vi "运维调试_总氮.vi"() -> ()   [LabVIEW 2016, in "斯坦道总氮.lvlib"]
uses:
  <vilib>/Utility/miscctls.llb/LVPointTypeDef.ctl
  <vilib>/Utility/config.llb/NI_LVConfig.lvlib
  <vilib>/ptbypt/NI_PtbyPt.lvlib
panel:
  out "一级权限":bool
  out "二级权限":bool
  out "输入密码":u32
  out "布尔":bool
  in  "流程固件":bool
  in  "仪器参数设置":bool
  in  "量程参数读取":T1
  in  "模块启用":bool
  in  "串口设置":bool
  in  "公式一键写入":bool
  in  "流程路径":path=path "C:/Users/STD/Documents/斯坦道流程文件/流程.xml"
  in  "曲线模型":cluster{"X^2":dbl, "X":dbl, "B":dbl}(xcontrol)
  out "字符串":string
  in  "质控参数设置":bool
  in  "自动测试量程配置":T2
  out "温度2":sgl
  out "温度1":sgl
  out "ADC":sgl
  out "固件版本号":string
  in  "数组":string[](array[string])
  in  "量程切换阈值写入":bool
  in  "量程切换阈值读取":bool
  in  "参数下拉列表":enum16{"总磷", "总氮"}(ring)=enum."总氮"
  in  "量程下拉列表":enum16{"低量程", "高量程"}(ring)
  in  "测量模式下拉列表":enum16{"水样测量", "零点核查", "跨度核查", "标样核查", "加标回收"}(ring)
  in  "公式":cluster{"X^2":dbl, "X":dbl, "b":dbl}
  in  "写公式":bool
  in  "读公式":bool
  in  "返回":bool
  in  "设置":bool
  out "序列号":string="序列号"
  out "测量数据":T3(xcontrol)
  out "集成报警信息":string
  out "定时启动":bool
  out "总磷总氮运行状态":T4(xcontrol)
  in  "停止":bool
  in  "手动启动":bool
  in  "单步测试":bool
  in  "总磷氨氮调试":u16[](xcontrol)
  out "F3":sgl format="%#.6f"
  out "F2":sgl format="%#.6f"
  out "F1":sgl format="%#.6f"
  out "F0":sgl format="%#.6f"
  out "多列列表框":i32(listbox)
  # "参数设置"
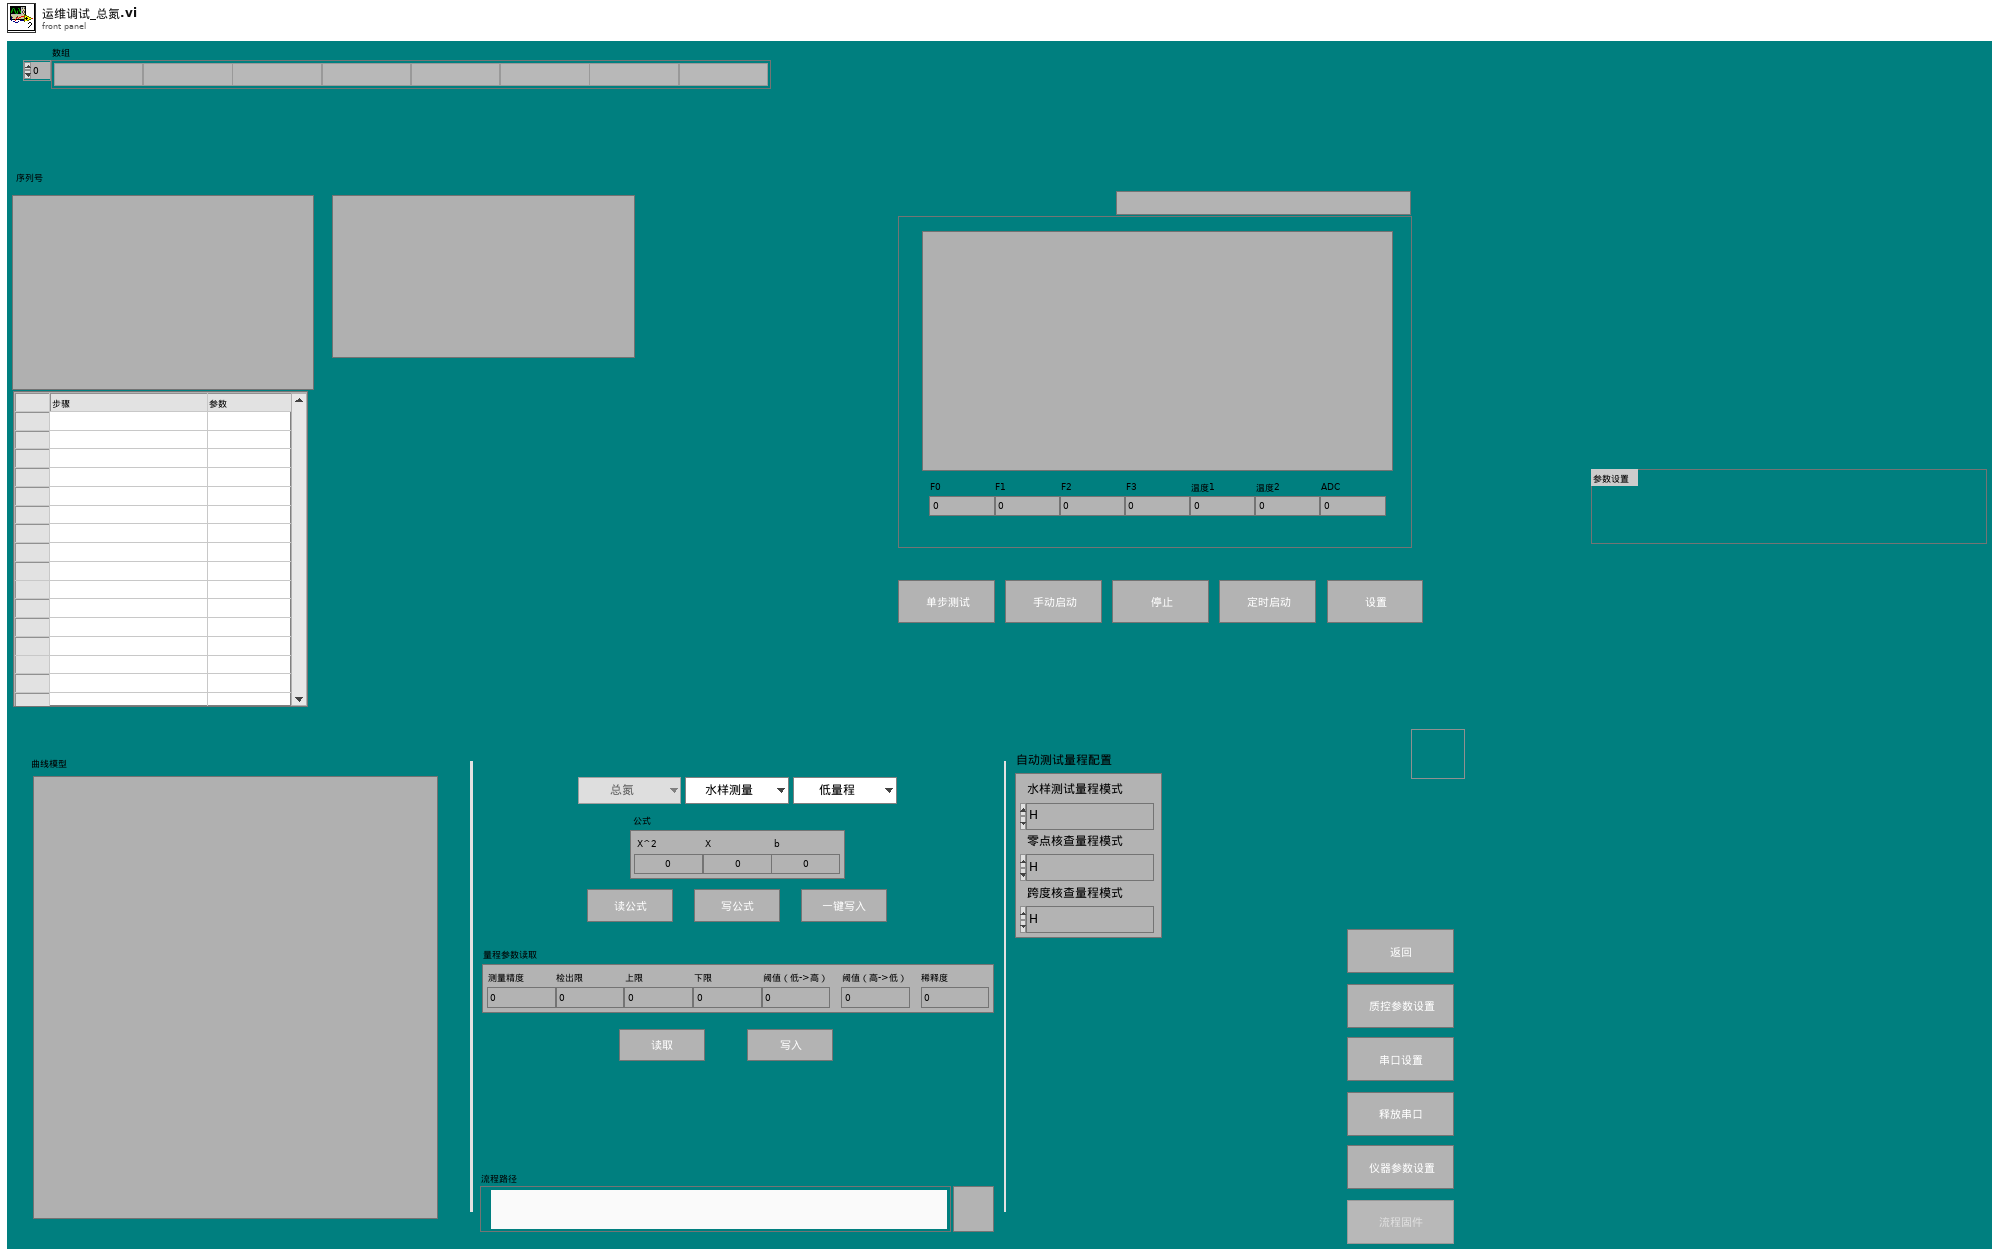
[diagram p1: front panel]
types:
  T1 = cluster{"测量精度":dbl, "检出限":dbl, "上限":dbl, "下限":dbl, "阈值（低->高）":dbl, "阈值（高->低）":dbl, "稀释度":dbl}
  T2 = cluster{"水样测试量程模式":enum16{"H", "L", "AUTO"}, "空白核查量程模式":enum16{"H", "L", "AUTO"}, "跨度核查量程模式":enum16{"H", "L", "AUTO"}}
  T3 = cluster{"flowid":u16, "测量精度":u16, "测量数据区":cluster{"因子编码":u32, "单位":u16, "标样参考值":sgl, "水样数据时间":timestamp, "水样实测值":sgl, "水样数据标识":string, "标样数据时间":timestamp, "标样实测值":sgl, "标样数据标识":string, "空白数据时间":timestamp, "空白实测值":sgl, "空白数据标识":string, "零点核查数据时间":timestamp, "零点核查实测值":sgl, "零点核查数据标识":string, "跨度核查数据时间":timestamp, "跨度核查实测值":sgl, "跨度核查数据标识":string, "加标回收数据时间":timestamp, "加标回收实测值":sgl, "加标回收数据标识":string, "平行样数据时间":timestamp, "平行样实测值":sgl, "平行样数据标识":string, "F0":sgl, "F1":sgl, "F2":sgl, "F3":sgl, "F4":sgl, "F5":sgl, "F6":sgl, "F7":sgl, "温度":sgl, "湿度":sgl, "X值":sgl, "fidrange":sgl}}
  T4 = cluster{"系统时间":timestamp, "工作状态":enum16{"空闲", "水样测试", "标样核查", "零点核查", "跨度核查", "空白测试", "平行样测试", "加标回收", "空白校准", "标样校准", "初始化（清洗）"}, "测量模式":enum16{"待机", "连续模式", "周期模式", "定点模式", "受控模式", "手动模式"}, "告警代码":u16, "故障代码":u16, "日志代码":u16, "软件版本":u16, "F0":sgl, "F1":sgl, "F2":sgl, "F3":sgl, "T":sgl, "H":sgl, "id":u16, "flowid":u16, "量程":u16, "总磷控温温度1":sgl, "营养盐控温温度2":sgl, "ADC":sgl}
  T5 = enum16{"启动测量", "标样核查", "零点核查", "跨度核查", "空白测试", "平行样测试", "加标回收", "空白校准", "标样校准", "初始化（清洗）", "停止测试", "仪器重启", "校时", "模式设置", "测量间隔设置"}
  T6 = cluster{"控制命令":enum16{"启动测量", "标样核查", "零点核查", "跨度核查", "空白测试", "平行样测试", "加标回收", "空白校准", "标样校准", "初始化（清洗）", "停止测试", "仪器重启", "校时", "模式设置", "测量间隔设置"}, "周期设置类型":enum16{"定点启动", "间隔启动"}, "定时功能启用":bool, "定时间隔":dbl, "24H周期设置":bool[], "零点核查时间":u16, "跨度核查时间":u16, "质控频次":enum16{"关闭", "每天", "星期一", "星期二", "星期三", "星期四", "星期五", "星期六", "星期日"}}
  T7 = enum16{"关闭", "每天", "星期一", "星期二", "星期三", "星期四", "星期五", "星期六", "星期日"}
  T8 = typedef "LVDateTimeRec.ctl" = cluster{"秒数的小数部分":dbl, "秒":i32, "分":i32, "时":i32, "日":i32, "月":i32, "年":i32, "天数（周）":i32, "天数（年）":i32, "DST":i32}
  T9 = enum16{"空闲", "水样测试", "标样核查", "零点核查", "跨度核查", "空白测试", "平行样测试", "加标回收", "空白校准", "标样校准", "初始化（清洗）"}
  T10 = enum32{"Bad", "Idle", "Run top level", "Running"}
  T11 = typedef "LVPointTypeDef.ctl" = cluster{"Horizontal":i16, "Vertical":i16}
  T12 = cluster{"因子编码":u32, "单位":u16, "标样参考值":sgl, "水样数据时间":timestamp, "水样实测值":sgl, "水样数据标识":string, "标样数据时间":timestamp, "标样实测值":sgl, "标样数据标识":string, "空白数据时间":timestamp, "空白实测值":sgl, "空白数据标识":string, "零点核查数据时间":timestamp, "零点核查实测值":sgl, "零点核查数据标识":string, "跨度核查数据时间":timestamp, "跨度核查实测值":sgl, "跨度核查数据标识":string, "加标回收数据时间":timestamp, "加标回收实测值":sgl, "加标回收数据标识":string, "平行样数据时间":timestamp, "平行样实测值":sgl, "平行样数据标识":string, "F0":sgl, "F1":sgl, "F2":sgl, "F3":sgl, "F4":sgl, "F5":sgl, "F6":sgl, "F7":sgl, "温度":sgl, "湿度":sgl, "X值":sgl, "fidrange":u16}
  T13 = typedef "NI_LVConfig.lvlib/Config Data RefNum.ctl" = refnum<k1>
  T14 = enum8{"Enabled", "Disabled", "Disabled and Grayed Out"}
  T15 = cluster{"启动模式":enum16{"跨度核查", "水样测量", "空白核查", "标样核查", "加标回收"}, "启动参数":u16, "量程":enum16{"低量程", "高量程"}}
  T16 = cluster{"时间标识":timestamp, "设备":string, "日志信息":string, "流程参数":string}
  T17 = cluster{"时间标识":timestamp, "设备":string, "日志信息":string}
  T18 = typedef "LVRowAndColumnUnsignedTypeDef.ctl" = cluster{"Row":u32, "Column":u32}
  T19 = cluster{"参数下拉列表":enum16{"总磷", "总氮"}, "测量模式下拉列表":enum16{"水样测量", "零点核查", "跨度核查", "标样核查", "加标回收"}, "量程下拉列表":enum16{"低量程", "高量程"}}
  T20 = cluster{"站号":u16, "量程切换":enum32{"H", "L", "AUTO"}, "控制命令":enum16{"启动测量", "标样核查", "零点核查", "跨度核查", "空白测试", "平行样测试", "加标回收", "空白校准", "标样校准", "初始化（清洗）", "停止测试", "仪器重启", "校时", "模式设置", "测量间隔设置"}, "模式设置":enum16{"待机", "连续模式", "周期模式", "定点模式", "受控模式", "手动模式"}, "测量间隔":u16}
  T21 = cluster{"跨度值":dbl, "零点标准液浓度":dbl, "跨度标准液浓度":dbl, "标准液标准浓度":dbl}
  T22 = cluster{"确定":bool, "跨度值":dbl, "零点标准液浓度":dbl, "跨度标准液浓度":dbl, "标准液标准浓度":dbl}
  T23 = cluster{"测量量程":dbl, "测量精度":dbl, "测量间隔":dbl, "消解温度":dbl, "消解时长":dbl, "空白校准时间":timestamp, "曲线截距":dbl, "曲线斜率":dbl, "测量检出限":dbl, "测量信号值":dbl, "线性相关系数":dbl, "二次多项式系数":dbl, "标样校准时间":timestamp, "单位":u16}
  T24 = cluster{"确定":bool, "测量量程":dbl, "测量精度":dbl, "测量间隔":dbl, "消解温度":dbl, "消解时长":dbl, "空白校准时间":timestamp, "曲线截距":dbl, "曲线斜率":dbl, "测量检出限":dbl, "测量信号值":dbl, "线性相关系数":dbl, "二次多项式系数":dbl, "标样校准时间":timestamp, "单位":u16}
  T25 = cluster{"控制命令":enum16{"启动测量", "标样核查", "零点核查", "跨度核查", "空白测试", "平行样测试", "加标回收", "空白校准", "标样校准", "初始化（清洗）", "停止测试", "仪器重启", "校时", "模式设置", "测量间隔设置"}, "周期设置类型":enum16{"定点启动", "间隔启动"}, "定时功能启用":bool, "定时间隔":dbl, "24H周期设置":bool[], "空白核查时间":u16, "跨度核查时间":u16, "质控频次":enum16{"关闭", "每天", "星期一", "星期二", "星期三", "星期四", "星期五", "星期六", "星期日"}}
  T26 = cluster{"测量精度":u16, "检出限":dbl, "上限":dbl, "下限":dbl, "阈值（低->高）":dbl, "阈值（高->低）":dbl, "稀释度":dbl}
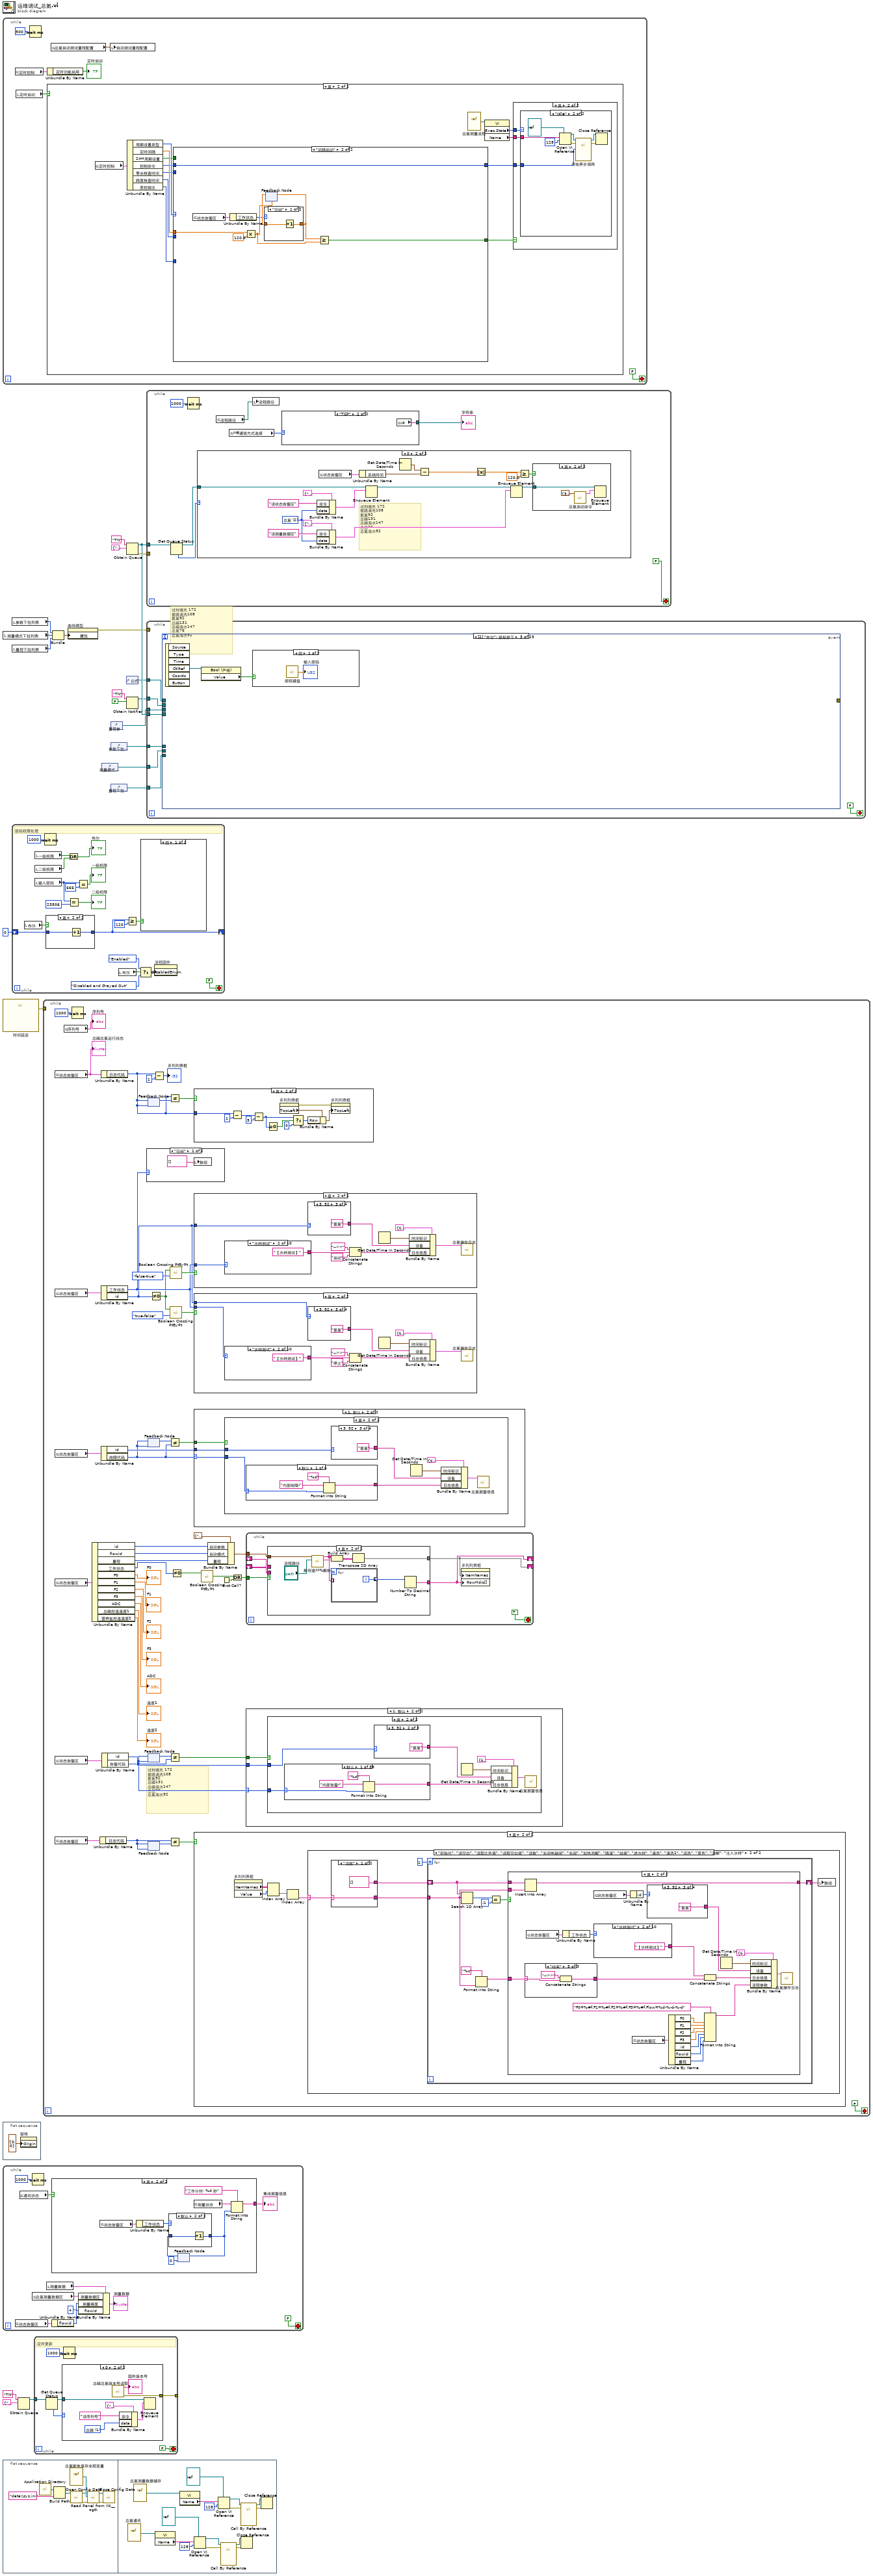
[diagram p0: block diagram]
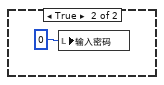
[diagram p2: hidden frame]
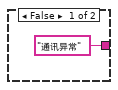
[diagram p5: hidden frame]
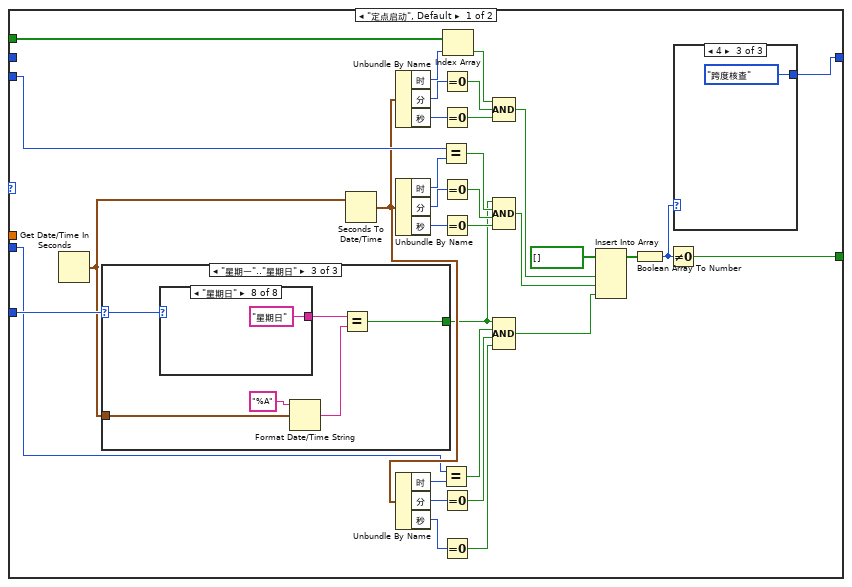
[diagram p8: hidden frame]
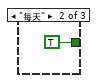
[diagram p10: hidden frame]
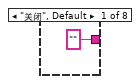
[diagram p11: hidden frame]
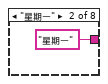
[diagram p12: hidden frame]
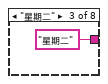
[diagram p13: hidden frame]
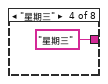
[diagram p14: hidden frame]
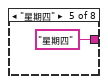
[diagram p15: hidden frame]
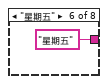
[diagram p16: hidden frame]
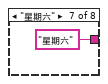
[diagram p17: hidden frame]
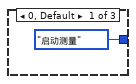
[diagram p18: hidden frame]
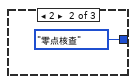
[diagram p19: hidden frame]
diagram:
  # "试剂填充 172 \n管路清洗108\n氨氮92\n总磷131\n总磷海水147\n总氮76\n总氮海水92"
  n1 = while {
    stop <- FALSE stop-if-true
    n2 = global read "总氮断电保存全局变量.vi" "定时控制"() -> (w24:T6)
    n3 = local read "定时启动"() -> (w26:bool)
    n4 = Wait (ms)(milliseconds to wait=u32 500 ("等待时间（毫秒）")) -> ()  [unwired: 1 out]
    n5 = Unbundle By Name(w24) -> ("定时功能启用"=→"定时启动":bool)
    n6 = case shown="真" w26 {
      frame False {
      }
      frame True {
        n7 = global read "总氮断电保存全局变量.vi" "定时控制"() -> (w41:T6)
        n8 = Unbundle By Name(w41) -> ("周期设置类型"=w37:enum16{"定点启动", "间隔启动"}, "定时间隔"=w36:dbl, "24H周期设置"=w35:bool[], "控制命令"=w34:T5, "零点核查时间"=w31:u16, "跨度核查时间"=w30:u16, "质控频次"=w29:T7)
        n9 = case shown="\"间隔启动\"" w37 {
          tunnel: w36 -> [_ w99]
          tunnel: w35 -> [w65 _]
          tunnel: [w43 w97] -> w32
          tunnel: w34 -> [_ w95]
          tunnel: [w69 w95] -> w33
          tunnel: w29 -> [w68 _]
          tunnel: w31 -> [w61 _]
          tunnel: w30 -> [w50 _]
          frame "定点启动", Default {
            n10 = Get Date/Time In Seconds() -> (seconds since 1Jan1904=w67:timestamp)
            n11 = case shown="\"星期一\"..\"星期日\"" w68 {
              selector: w68 -> [_ _ w79]
              tunnel: w67 -> [_ _ w80]
              tunnel: [_ TRUE w76] -> w49
              frame "关闭", Default {
              }
              frame "每天" {
              }
              frame "星期一".."星期日" {
                n12 = case shown="\"星期日\"" w79 {
                  tunnel: ["" ("时间格式字符串(%c)") "星期一" ("时间格式字符串(%c)") "星期二" ("时间格式字符串(%c)") "星期三" ("时间格式字符串(%c)") "星期四" ("时间格式字符串(%c)") "星期五" ("时间格式字符串(%c)") "星期六" ("时间格式字符串(%c)") "星期日" ("时间格式字符串(%c)")] -> w78
                  frame "关闭", Default {
                  }
                  frame "星期一" {
                  }
                  frame "星期二" {
                  }
                  frame "星期三" {
                  }
                  frame "星期四" {
                  }
                  frame "星期五" {
                  }
                  frame "星期六" {
                  }
                  frame "星期日" {
                  }
                }
                n13 = Format Date/Time String(time format string (%c)="%A" ("时间格式字符串(%c)"), seconds (now)=w80) -> (date/time string=w77:string)  [unwired: 1 in]
                n14 = Equal?(x=w78, y=w77) -> (x = y?=w76:bool)
              }
            }
            n15 = Seconds To Date/Time(time stamp (now)=w67) -> (date time rec=w51:T8)  [unwired: 1 in]
            n16 = Unbundle By Name(w51) -> ("时"=w74:i32, "分"=w72:i32, "秒"=w73:i32)
            n17 = Unbundle By Name(w51) -> ("时"=w62:i32, "分"=w64:i32, "秒"=w63:i32)
            n18 = Unbundle By Name(w51) -> ("时"=w54:i32, "分"=w52:i32, "秒"=w53:i32)
            n19 = Equal?(x=w61, y=w62) -> (x = y?=w60:bool)
            n20 = Equal?(x=w50, y=w54) -> (x = y?=w55:bool)
            n21 = Equal To 0?(x=w72) -> (x = 0?=w71:bool)
            n22 = Equal To 0?(x=w73) -> (x = 0?=w70:bool)
            n23 = Equal To 0?(x=w64) -> (x = 0?=w59:bool)
            n24 = Equal To 0?(x=w63) -> (x = 0?=w58:bool)
            n25 = Equal To 0?(x=w52) -> (x = 0?=w56:bool)
            n26 = Equal To 0?(x=w53) -> (x = 0?=w57:bool)
            n27 = Index Array(array=w65, index=w74) -> (element=w66:bool)
            n28 = Compound Arithmetic op=AND ("复合运算")(w66, w71, w70) -> (w47:bool)
            n29 = Compound Arithmetic op=AND ("复合运算")(w49, w60, w59, w58) -> (w46:bool)
            n30 = Compound Arithmetic op=AND ("复合运算")(w49, w55, w56, w57) -> (w45:bool)
            n31 = Insert Into Array(array=bool[] [], new element #1=w47, new element #2=w46, new element #3=w45) -> (w44:bool[])  [unwired: 1 in]
            n32 = Boolean Array To Number(Boolean array=w44) -> (number=w42:u32)
            n33 = Not Equal To 0?(x=w42) -> (x != 0?=w43:bool)
            n34 = case shown="4" w42 {
              tunnel: [T5."启动测量" ("控制命令") T5."零点核查" ("控制命令") T5."跨度核查" ("控制命令")] -> w69
              frame 0, Default {
              }
              frame 2 {
              }
              frame 4 {
              }
            }
          }
          frame "间隔启动" {
            n35 = global read "VAR总氮全局变量.vi" "状态告警区"() -> (w94:T4)
            n36 = Unbundle By Name(w94) -> ("工作状态"=w93:T9)
            n37 = Multiply(x=w99, y=120.0) -> (x*y=w96:dbl)
            n38 = feedback #1(w96) -> (w101:dbl)
            n39 = case shown="\"空闲\"" w93 {
              tunnel: w101 -> [w103 _]
              tunnel: [w102 _] -> w100
              frame "空闲" {
                n40 = Increment(x=w103) -> (x+1=w102:dbl)
              }
              frame "水样测试", Default {
              }
            }
            n41 = feedback-in #1(w100) -> ()
            n42 = Greater Or Equal?(x=w100, y=w96) -> (x >= y?=w97:bool)
          }
        }
        n43 = vi-ref "总氮测量流程.vi"() -> (w40:refnum<vi>)
        n44 = property class="VI"(reference=w40) -> ("Exec.State"=w38:T10, "Name"=w39:string)  [unwired: 1 in, 2 out]
        n45 = case shown="真" w32 {
          tunnel: w39 -> [_ w106]
          tunnel: w33 -> [_ w105]
          tunnel: w38 -> [_ w104]
          frame False {
          }
          frame True {
            n46 = case shown="\"Idle\"" w104 {
              tunnel: w106 -> [_ w110]
              tunnel: w105 -> [_ w108]
              frame "Bad", Default {
              }
              frame "Idle" {
                n47 = Open VI Reference(type specifier VI Refnum (for type only)=refnum<vi> refnum, vi path=w110, options=128 ("选项")) -> (vi reference=w111:refnum<vi>, error out=w112:errorcluster)  [unwired: 3 in]
                n48 = call-by-ref "开始异步调用"(reference=w111, error in=w112, "控制命令"=w108) -> (reference out=w113:refnum<vi>, error out=w114:errorcluster)  [unwired: 11 in]
                n49 = Close Reference(reference=w113, error in (no error)=w114) -> ()  [unwired: 1 out]
              }
            }
          }
        }
      }
    }
    n50 = global read "总氮断电保存全局变量.vi" "总氮自动测试量程配置"() -> (w25:T2)
    n51 = local write "自动测试量程配置"(w25) -> ()
  }
  n52 = local read "测量模式下拉列表"() -> (w4:enum16{"水样测量", "零点核查", "跨度核查", "标样核查", "加标回收"})
  n53 = call "时间延迟"() -> ("error out"=w14:errorcluster)  [unwired: 11 in]
  n54 = flat-sequence {
    frame #0 {
      n55 = property on="窗格" class="Pane"("Origin"=T11 {"Horizontal"=0, "Vertical"=0} ("原点")) -> ()  [unwired: 2 in, 2 out]
    }
  }
  n56 = while {
    stop <- FALSE stop-if-true
    n57 = global read "VAR总氮全局变量.vi" "状态告警区"() -> (w121:T4)
    n58 = global read "VAR总氮全局变量.vi" "通讯状态"() -> (w123:bool)
    n59 = Wait (ms)(milliseconds to wait=u32 1000 ("等待时间（毫秒）")) -> ()  [unwired: 1 out]
    n60 = global read "VAR总氮全局变量.vi" "总氮测量数据区"() -> (w117:T12)
    n61 = local read "测量数据"() -> (w116:T3)
    n62 = case shown="真" w123 {
      tunnel: ["通讯异常" ("集成报警信息") w128] -> w122
      frame False {
      }
      frame True {
        n63 = global read "VAR总氮全局变量.vi" "状态告警区"() -> (w134:T4)
        n64 = Unbundle By Name(w134) -> ("工作状态"=w133:T9)
        n65 = feedback #2(0) -> (w131:i32)
        n66 = case shown="默认" w133 {
          tunnel: w131 -> [_ w136]
          tunnel: [_ w135] -> w129
          frame "空闲" {
          }
          frame Default {
            n67 = Increment(x=w136) -> (x+1=w135:i32)
          }
        }
        n68 = feedback-in #2(w129) -> ()
        n69 = global read "VAR总氮全局变量.vi" "测量状态"() -> (w127:string)
        n70 = Format Into String(format string="工作计时: %d 秒" ("格式字符串"), initial string=w127, w129) -> (resulting string=w128:string)  [unwired: 1 in, 1 out]
      }
    }
    "集成报警信息" <- w122
    n71 = Unbundle By Name(w121) -> ("flowid"=w120:u16)
    n72 = Bundle By Name(cluster=w116, "测量数据区"=w117, "测量精度"=u16 4, "flowid"=w120) -> (→"测量数据":T3)
  }
  n73 = flat-sequence {
    frame #0 {
      n74 = call <vilib>:"Application Directory.vi"() -> ("Application Directory"=w144:path)
      n75 = Build Path(base path=w144, name or relative path="data\\sys.ini" ("名称或相对路径")) -> (appended path=w142:path)
      n76 = vi-ref "总氮断电保存全局变量.vi"() -> (w140:refnum<vi>)
      n77 = call <vilib>:"Open Config Data.vi"("configuration file path"=w142) -> ("error out"=w138:errorcluster, "refnum"=w141:T13)  [unwired: 8 in, 1 out]
      n78 = call <userlib>:"Read Panel from INI__ogtk.vi"("error in (no error)"=w138, "VI ref"=w140, "refnum"=w141) -> ("error out"=w137:errorcluster, "refnum out"=w139:T13)  [unwired: 7 in]
      n79 = call <vilib>:"Close Config Data.vi"("error in (no error)"=w137, "refnum"=w139) -> ()  [unwired: 8 in, 2 out]
    }
    frame #1 {
      n80 = vi-ref "总氮通讯.vi"() -> (w160:refnum<vi>)
      n81 = vi-ref "总氮测量数据储存.vi"() -> (w152:refnum<vi>)
      n82 = property class="VI"(reference=w160) -> ("Name"=w159:string)  [unwired: 1 in, 2 out]
      n83 = property class="VI"(reference=w152) -> ("Name"=w145:string)  [unwired: 1 in, 2 out]
      n84 = Open VI Reference(type specifier VI Refnum (for type only)=refnum<vi> refnum, vi path=w159, options=128 ("选项")) -> (vi reference=w157:refnum<vi>, error out=w155:errorcluster)  [unwired: 3 in]
      n85 = Open VI Reference(type specifier VI Refnum (for type only)=refnum<vi> refnum, vi path=w145, options=128 ("选项")) -> (vi reference=w147:refnum<vi>, error out=w149:errorcluster)  [unwired: 3 in]
      n86 = call-by-ref "?"(reference=w157, error in=w155) -> (reference out=w153:refnum<vi>, error out=w154:errorcluster)  [unwired: 12 in]
      n87 = call-by-ref "?"(reference=w147, error in=w149) -> (reference out=w151:refnum<vi>, error out=w150:errorcluster)  [unwired: 12 in]
      n88 = Close Reference(reference=w153, error in (no error)=w154) -> ()  [unwired: 1 out]
      n89 = Close Reference(reference=w151, error in (no error)=w150) -> ()  [unwired: 1 out]
    }
  }
  n90 = local read "参数下拉列表"() -> (w5:enum16{"总磷", "总氮"})
  n91 = local read "量程下拉列表"() -> (w3:enum16{"低量程", "高量程"})
  n92 = while {
    shift-right: [w167] -> _
    shift-left: u32 0 ("等待时间（毫秒）") -> [w168]
    stop <- FALSE stop-if-true
    # "密码权限处理"
    n93 = local read "布尔"() -> (w169:bool)
    n94 = local read "一级权限"() -> (w171:bool)
    n95 = local read "二级权限"() -> (w172:bool)
    n96 = local read "输入密码"() -> (w175:u32)
    n97 = Wait (ms)(milliseconds to wait=u32 1000 ("等待时间（毫秒）")) -> ()  [unwired: 1 out]
    n98 = case shown="真" w169 {
      tunnel: w168 -> [_ w182]
      tunnel: [_ w181] -> w167
      frame False {
      }
      frame True {
        n99 = Increment(x=w182) -> (x+1=w181:u32)
      }
    }
    n100 = Or(x=w171, y=w172) -> (x .or. y?=→"布尔":bool)
    n101 = Equal?(x=w175, y=u32 23506) -> (x = y?=→"二级权限":bool)
    n102 = Equal?(x=w175, y=u32 666) -> (x = y?=→"一级权限":bool)
    n103 = local read "布尔"() -> (w164:bool)
    n104 = Greater Or Equal?(x=w167, y=u32 120) -> (x >= y?=w165:bool)
    n105 = Select(t=T14."Enabled" ("禁用"), s=w164, f=T14."Disabled and Grayed Out") -> (s? t:f=w162:T14)
    n106 = case shown="假" w165 {
      frame False {
      }
      frame True {
        n107 = local write "输入密码"(u32 0 ("输入密码")) -> ()
      }
    }
    n108 = property on="流程固件" class="Bool"("DisabledEnum"=w162) -> ()  [unwired: 2 in, 2 out]
  }
  n109 = Obtain Queue(name (unnamed)="TN" ("名称（未命名）"), element data type=cluster{"命令":string, "data":variant} {"命令"="", "data"=variant}) -> (queue out=w11:refnum<queue>)  [unwired: 3 in, 2 out]
  n110 = while {
    tunnel: w11 -> [w187]
    tunnel: [w185] -> _
    stop <- FALSE stop-if-true
    # "定时更新"
    n111 = Get Queue Status(queue=w187) -> (queue out=w184:refnum<queue>, # elements in queue=w183:i32)  [unwired: 2 in, 6 out]
    n112 = case shown="0" w183 {
      tunnel: [_ w190] -> w185
      tunnel: w184 -> [_ w189]
      frame Default {
      }
      frame 0 {
        w193 = u16 1 items=["总磷"=1, "氨氮"=3] ("站号")
        n113 = call "总磷总氮版本号读取.vi"() -> ("error out"=w190:errorcluster, "固件版本号"=→"固件版本号":string)  [unwired: 10 in]
        n114 = Bundle By Name(cluster=cluster{"命令":string, "data":variant} {"命令"="", "data"=variant} ("元素"), "命令"="读序列号", "data"=w193) -> (w192:cluster{"命令":string, "data":variant})
        n115 = Enqueue Element(queue=w189, element=w192) -> ()  [unwired: 2 in, 3 out]
      }
    }
    n116 = Wait (ms)(milliseconds to wait=u32 1000 ("等待时间（毫秒）")) -> ()  [unwired: 1 out]
  }
  n117 = while {
    tunnel: w14 -> [_]
    stop <- FALSE stop-if-true
    # "试剂填充 172 \n管路清洗108\n氨氮92\n总磷131\n总磷海水147\n总氮76\n总氮海水92"
    n118 = global read "VAR总氮全局变量.vi" "状态告警区"() -> (w229:T4)
    "总磷总氮运行状态" <- w229
    n119 = global read "VAR总氮全局变量.vi" "状态告警区"() -> (w216:T4)
    n120 = global read "VAR总氮全局变量.vi" "状态告警区"() -> (w221:T4)
    n121 = global read "VAR总氮全局变量.vi" "状态告警区"() -> (w237:T4)
    n122 = global read "VAR总氮全局变量.vi" "状态告警区"() -> (w226:T4)
    n123 = global read "VAR总氮全局变量.vi" "状态告警区"() -> (w214:T4)
    n124 = global read "VAR总氮全局变量.vi" "序列号"() -> (→"序列号":string)
    n125 = Wait (ms)(milliseconds to wait=u32 1000 ("等待时间（毫秒）")) -> ()  [unwired: 1 out]
    n126 = Unbundle By Name(w237) -> ("id"=w234:u16, "flowid"=w236:u16, "量程"=w235:u16, "工作状态"=w204:T9, "F0"=→"F0":sgl, "F1"=→"F1":sgl, "F2"=→"F2":sgl, "F3"=→"F3":sgl, "ADC"=→"ADC":sgl, "总磷控温温度1"=→"温度1":sgl, "营养盐控温温度2"=→"温度2":sgl)
    n127 = Unbundle By Name(w214) -> ("日志代码"=w213:u16)
    n128 = Unbundle By Name(w229) -> ("日志代码"=w210:u16)
    n129 = Unbundle By Name(w216) -> ("工作状态"=w200:T9, "id"=w199:u16)
    n130 = Unbundle By Name(w221) -> ("id"=w220:u16, "故障代码"=w217:u16)
    n131 = Unbundle By Name(w226) -> ("id"=w225:u16, "告警代码"=w222:u16)
    n132 = case shown="\"空闲\"" w200 {
      frame "空闲" {
        n133 = local write "数组"(string[] [] ("数组")) -> ()
      }
      frame "水样测试", Default {
      }
    }
    n134 = feedback-in #3(w210) -> ()
    n135 = feedback #3(w210) -> (w242:u16)
    n136 = feedback #4(w217) -> (w218:u16)
    n137 = feedback-in #4(w217) -> ()
    n138 = feedback #5(w222) -> (w223:u16)
    n139 = feedback-in #5(w222) -> ()
    n140 = feedback #6(w213) -> (w215:u16)
    n141 = feedback-in #6(w213) -> ()
    n142 = Not Equal To 0?(x=w199) -> (x != 0?=w197:bool)
    n143 = Subtract(x=w210, y=1) -> (x-y=→"多列列表框":i32)
    n144 = Not Equal?(x=w210, y=w242) -> (x != y?=w241:bool)
    n145 = Not Equal?(x=w218, y=w217) -> (x != y?=w219:bool)
    n146 = Not Equal?(x=w223, y=w222) -> (x != y?=w224:bool)
    n147 = Not Equal?(x=w213, y=w215) -> (x != y?=w212:bool)
    n148 = call <vilib>:"Boolean Crossing PtByPt.vi"("direction"=enum16{"either", "false-true", "true-false"}."false-true", "input"=w197) -> ("crossing"=w202:bool)  [unwired: 1 in]
    n149 = call <vilib>:"Boolean Crossing PtByPt.vi"("direction"=enum16{"either", "false-true", "true-false"}."true-false", "input"=w197) -> ("crossing"=w196:bool)  [unwired: 1 in]
    n150 = Not Equal To 0?(x=w204) -> (x != 0?=w239:bool)
    n151 = case shown="真" w241 {
      tunnel: w210 -> [_ w452]
      frame False {
      }
      frame True {
        n152 = Subtract(x=w452, y=1) -> (x-y=w450:i32)
        n153 = Subtract(x=w450, y=5) -> (x-y=w454:i32)
        n154 = Greater Or Equal To 0?(x=w454) -> (x >= 0?=w453:bool)
        n155 = property on="多列列表框" class="MCListbox (严格)"() -> (error out=w458:errorcluster, "TopLeft"=w459:T18)  [unwired: 2 in, 1 out]
        n156 = Select(t=w454, s=w453, f=0) -> (s? t:f=w455:i32)
        n157 = Bundle By Name(cluster=w459, "Row"=w455) -> (w460:T18)
        n158 = property on="多列列表框" class="MCListbox (严格)"(error in=w458, "TopLeft"=w460) -> ()  [unwired: 1 in, 2 out]
      }
    }
    n159 = case shown="真" w202 {
      tunnel: w199 -> [_ w270]
      tunnel: w200 -> [_ w269]
      frame False {
      }
      frame True {
        n160 = case shown="\"水样测试\"" w269 {
          tunnel: [_ "【水样测试】" ("字符串") "【标样核查】" ("字符串") "【零点核查】" ("字符串") "【跨度核查】" ("字符串") "【空白测试】" ("字符串") "【平行样测试】" ("字符串") "【加标回收】" ("字符串") "【空白校准】" ("字符串") "【标样校准】" ("字符串")] -> w275
          frame "空闲", Default {
          }
          frame "水样测试" {
          }
          frame "标样核查" {
          }
          frame "零点核查" {
          }
          frame "跨度核查" {
          }
          frame "空白测试" {
          }
          frame "平行样测试" {
          }
          frame "加标回收" {
          }
          frame "空白校准" {
          }
          frame "标样校准" {
          }
        }
        n161 = case shown="3, 92" w270 {
          tunnel: [_ "总磷" ("table输入") "氨氮" ("table输入") "总氮" ("table输入")] -> w272
          frame Default {
          }
          frame 1, 131 {
          }
          frame 3, 92 {
          }
          frame 2, 76 {
          }
        }
        n162 = Concatenate Strings("-->>" ("字符串"), w275, "启动" ("字符串")) -> (w276:string)
        n163 = Get Date/Time In Seconds() -> (seconds since 1Jan1904=w273:timestamp)
        n164 = Bundle By Name(cluster=T16 {"时间标识"=timestamp(0 s since 1904-01-01), "设备"="", "日志信息"="", "流程参数"=""} ("data in"), "时间标识"=w273, "设备"=w272, "日志信息"=w276) -> (w271:T16)
        n165 = call "总氮操作日志.vi"("data in"=w271) -> ()  [unwired: 11 in]
      }
    }
    n166 = case shown="真" w196 {
      tunnel: w199 -> [_ w248]
      tunnel: w200 -> [_ w247]
      frame False {
      }
      frame True {
        n167 = case shown="\"水样测试\"" w247 {
          tunnel: [_ "【水样测试】" ("字符串") "【标样核查】" ("字符串") "【零点核查】" ("字符串") "【跨度核查】" ("字符串") "【空白测试】" ("字符串") "【平行样测试】" ("字符串") "【加标回收】" ("字符串") "【空白校准】" ("字符串") "【标样校准】" ("字符串")] -> w253
          frame "空闲", Default {
          }
          frame "水样测试" {
          }
          frame "标样核查" {
          }
          frame "零点核查" {
          }
          frame "跨度核查" {
          }
          frame "空白测试" {
          }
          frame "平行样测试" {
          }
          frame "加标回收" {
          }
          frame "空白校准" {
          }
          frame "标样校准" {
          }
        }
        n168 = case shown="3, 92" w248 {
          tunnel: [_ "总磷" ("table输入") "氨氮" ("table输入") "总氮" ("table输入")] -> w250
          frame Default {
          }
          frame 1, 131 {
          }
          frame 3, 92 {
          }
          frame 2, 76 {
          }
        }
        n169 = Concatenate Strings("-->>" ("字符串"), w253, "停止" ("字符串")) -> (w254:string)
        n170 = Get Date/Time In Seconds() -> (seconds since 1Jan1904=w251:timestamp)
        n171 = Bundle By Name(cluster=T16 {"时间标识"=timestamp(0 s since 1904-01-01), "设备"="", "日志信息"="", "流程参数"=""} ("data in"), "时间标识"=w251, "设备"=w250, "日志信息"=w254) -> (w249:T16)
        n172 = call "总氮操作日志.vi"("data in"=w249) -> ()  [unwired: 11 in]
      }
    }
    n173 = case shown="1, 默认" w217 {
      selector: w217 -> [_ w357]
      tunnel: w220 -> [_ w358]
      tunnel: w219 -> [_ w356]
      frame 0 {
      }
      frame 1, Default {
        n174 = case shown="真" w356 {
          tunnel: w358 -> [_ w365]
          tunnel: w357 -> [_ w360]
          frame False {
          }
          frame True {
            n175 = case shown="默认" w360 {
              selector: w360 -> [w367 _ _ _ _ _]
              tunnel: [w366 "无故障" "电机故障" "温度故障" "通讯故障" "滴定故障"] -> w359
              frame Default {
                n176 = Format Into String(format string="%d" ("格式字符串"), initial string="内部故障-" ("工作状态"), w367) -> (resulting string=w366:string)  [unwired: 1 in, 1 out]
              }
              frame 0 {
              }
              frame 1 {
              }
              frame 2 {
              }
              frame 3 {
              }
              frame 4 {
              }
            }
            n177 = case shown="3, 92" w365 {
              tunnel: [_ "总磷" ("table输入") "氨氮" ("table输入") "总氮" ("table输入")] -> w361
              frame Default {
              }
              frame 1, 131 {
              }
              frame 3, 92 {
              }
              frame 2, 76 {
              }
            }
            n178 = Get Date/Time In Seconds() -> (seconds since 1Jan1904=w362:timestamp)
            n179 = Bundle By Name(cluster=T17 {"时间标识"=timestamp(0 s since 1904-01-01), "设备"="", "日志信息"=""} ("data in"), "时间标识"=w362, "设备"=w361, "日志信息"=w359) -> (w363:T17)
            n180 = call "总氮报警信息.vi"("data in"=w363) -> ()  [unwired: 10 in, 1 out]
          }
        }
      }
    }
    n181 = case shown="真" w212 {
      frame False {
      }
      frame True {
        n182 = property on="多列列表框" class="MCListbox (严格)"() -> ("ItemNames"=w292:string[][], "Value"=w293:i32)  [unwired: 2 in, 2 out]
        n183 = Index Array(array=w292, index (row)=w293) -> (element=w291:string[])  [unwired: 1 in]
        n184 = Index Array(array=w291) -> (element=w290:string)  [unwired: 1 in]
        n185 = case shown="\"初始化\", \"读空白\", \"读取比色值\", \"读取空白值\", \"读数\", \"关闭电磁阀\", \"关阀\", \"加热消解\", \"降温\", \"结束\", \"进水样\", \"清洗\", \"清洗1\", \"润洗\", \"显色\", \"消解\", \"注入水样\"" w290 {
          selector: w290 -> [_ w296]
          frame Default {
          }
          frame "初始化", "读空白", "读取比色值", "读取空白值", "读数", "关闭电磁阀", "关阀", "加热消解", "降温", "结束", "进水样", "清洗", "清洗1", "润洗", "显色", "消解", "注入水样" {
            n186 = case shown="\"读数\"" w296 {
              selector: w296 -> [w300 w302]
              tunnel: [w300 w302] -> w295
              tunnel: [string[] [] ("数组") "数组"] -> w294
              frame "读数" {
              }
              frame Default {
              }
            }
            n187 = for {
              N: 1 -> [_]
              tunnel: w295 -> [w304]
              shift-right: [w303] -> w297
              shift-left: w294 -> [w305]
              n188 = Search 1D Array(1D array=w305, element=w304) -> (index of element=w308:i32)  [unwired: 1 in]
              n189 = Format Into String(format string="%s" ("格式字符串"), w304) -> (resulting string=w309:string)  [unwired: 2 in, 1 out]
              n190 = Equal?(x=w308, y=-1) -> (x = y?=w306:bool)
              n191 = case shown="真" w306 {
                tunnel: w309 -> [_ w317]
                tunnel: w305 -> [w311 w321]
                tunnel: w304 -> [_ w320]
                tunnel: [w311 w319] -> w303
                frame False {
                }
                frame True {
                  n192 = Insert Into Array(array=w321, new element=w320) -> (w319:string[])  [unwired: 1 in]
                  n193 = case shown="\"结束\"" w317 {
                    selector: w317 -> [w346 w349 w352]
                    tunnel: [w346 w348 w351] -> w313
                    frame Default {
                    }
                    frame "初始化" {
                      n194 = Concatenate Strings("-->>" ("字符串"), w349) -> (w348:string)
                    }
                    frame "结束" {
                      n195 = Concatenate Strings("-->>" ("字符串"), w352) -> (w351:string)
                    }
                  }
                  n196 = global read "VAR总氮全局变量.vi" "状态告警区"() -> (w316:T4)
                  n197 = Unbundle By Name(w316) -> ("工作状态"=w315:T9)
                  n198 = global read "VAR总氮全局变量.vi" "状态告警区"() -> (w336:T4)
                  n199 = case shown="\"水样测试\"" w315 {
                    tunnel: [_ "【水样测试】" ("字符串") "【标样核查】" ("字符串") "【零点核查】" ("字符串") "【跨度核查】" ("字符串") "【空白测试】" ("字符串") "【平行样测试】" ("字符串") "【加标回收】" ("字符串") "【空白校准】" ("字符串") "【标样校准】" ("字符串")] -> w314
                    frame "空闲", Default {
                    }
                    frame "水样测试" {
                    }
                    frame "标样核查" {
                    }
                    frame "零点核查" {
                    }
                    frame "跨度核查" {
                    }
                    frame "空白测试" {
                    }
                    frame "平行样测试" {
                    }
                    frame "加标回收" {
                    }
                    frame "空白校准" {
                    }
                    frame "标样校准" {
                    }
                  }
                  n200 = Unbundle By Name(w336) -> ("id"=w335:u16)
                  n201 = global read "VAR总氮全局变量.vi" "状态告警区"() -> (w331:T4)
                  n202 = case shown="3, 92" w335 {
                    tunnel: [_ "总磷" ("table输入") "氨氮" ("table输入") "总氮" ("table输入")] -> w333
                    frame Default {
                    }
                    frame 1, 131 {
                    }
                    frame 3, 92 {
                    }
                    frame 2, 76 {
                    }
                  }
                  n203 = Unbundle By Name(w331) -> ("F0"=w328:sgl, "F1"=w327:sgl, "F2"=w326:sgl, "F3"=w325:sgl, "id"=w324:u16, "flowid"=w323:u16, "量程"=w322:u16)
                  n204 = Concatenate Strings(w314, w313) -> (w312:string)
                  n205 = Format Into String(format string="F0=%#f,F1=%#f,F2=%#f,F3=%#f,Flow=%d-%-d-%-d" ("格式字符串"), w328, w327, w326, w325, w324, w323, w322) -> (resulting string=w329:string)  [unwired: 2 in, 1 out]
                  n206 = Get Date/Time In Seconds() -> (seconds since 1Jan1904=w332:timestamp)
                  n207 = Bundle By Name(cluster=T16 {"时间标识"=timestamp(0 s since 1904-01-01), "设备"="", "日志信息"="", "流程参数"=""} ("data in"), "时间标识"=w332, "设备"=w333, "日志信息"=w312, "流程参数"=w329) -> (w334:T16)
                  n208 = call "总氮操作日志.vi"("data in"=w334) -> ()  [unwired: 11 in]
                }
              }
            }
            n209 = local write "数组"(w297) -> ()
          }
        }
      }
    }
    n210 = call <vilib>:"Boolean Crossing PtByPt.vi"("input"=w239) -> ("crossing"=w203:bool)  [unwired: 2 in]
    n211 = Bundle By Name(cluster=T15 {"启动模式"=enum."跨度核查", "启动参数"=1, "量程"=enum."低量程"} ("参数簇"), "启动参数"=w234, "启动模式"=w236, "量程"=w235) -> (w228:T15)
    n212 = First Call?() -> (First Call?: T/F=w240:bool)
    n213 = Or(x=w203, y=w240) -> (x .or. y?=w238:bool)
    n214 = while {
      tunnel: w238 -> [w438]
      tunnel: w228 -> [w437]
      shift-right: [w432] -> _
      shift-left: _ -> [w434]
      shift-right: [w433] -> _
      shift-left: _ -> [w435]
      stop <- TRUE stop-if-true
      n215 = case shown="真" w438 {
        tunnel: [w440 w448] -> w433
        tunnel: [w439 w447] -> w432
        tunnel: w437 -> [_ w442]
        tunnel: w435 -> [w440 _]
        tunnel: w434 -> [w439 _]
        frame False {
        }
        frame True {
          n216 = call "斯坦道XML解析.vi"("添加的路径"="流程路径", "参数簇"=w442) -> ("步骤时间"=w443:string[], "步骤名"=w445:string[])  [unwired: 8 in]
          n217 = Build Array(w445, w443) -> (w444:string[][])
          n218 = for {
            tunnel: w445 -> [_] mode=indexing
            tunnel: [w449] -> w446 mode=indexing
            i -> [w449]
          }
          n219 = Transpose 2D Array(2D array=w444) -> (transposed array=w447:string[][])
          n220 = Number To Decimal String(number=w446) -> (decimal integer string=w448:string[])  [unwired: 1 in]
        }
      }
      n221 = property on="多列列表框" class="MCListbox (严格)"("ItemNames"=w432, "RowHdrs[]"=w433) -> ()  [unwired: 2 in, 2 out]
    }
    n222 = case shown="1, 默认" w222 {
      selector: w222 -> [_ w379]
      tunnel: w225 -> [_ w380]
      tunnel: w224 -> [_ w378]
      frame 0 {
      }
      frame 1, Default {
        n223 = case shown="真" w378 {
          tunnel: w380 -> [_ w387]
          tunnel: w379 -> [_ w381]
          frame False {
          }
          frame True {
            n224 = case shown="默认" w381 {
              selector: w381 -> [w389 _ _ _ _ _ _ _ _ _ _ _ _ _ _ _ _ _ _ _ _ _ _ _ _ _ _ _ _ _ _ _ _ _ _ _ _ _]
              tunnel: [w388 "无告警" "缺试剂告警" "缺水样告警" "缺蒸馏水告警" "缺标液告警" "仪表漏液告警" "标定异常告警" "超量程告警" "加热异常" "低试剂预警" "超上限告警" "超下限告警" "仪表内部其他异常" "滴定异常告警" "电极异常告警" "量程切换告警" "参数设置告警" "PH电极电位异常" "电导率电极异常" "浊度光度异常" "溶解氧电极异常" "溶解氧光强异常" "温度异常告警" "PH异常告警" "溶解氧异常告警" "电导率异常告警" "浊度异常告警" "叶绿素异常告警" "藻密度异常告警" "蓝绿藻异常告警" "ORP异常告警" "氨氮异常告警" "清洁刷异常告警" "SD卡异常告警" "蓝牙异常告警" "WiFi异常告警" "流程异常告警"] -> w382
              frame Default {
                n225 = Format Into String(format string="%d" ("格式字符串"), initial string="内部告警-" ("工作状态"), w389) -> (resulting string=w388:string)  [unwired: 1 in, 1 out]
              }
              frame 0 {
              }
              frame 1 {
              }
              frame 2 {
              }
              frame 3 {
              }
              frame 4 {
              }
              frame 5 {
              }
              frame 6 {
              }
              frame 7 {
              }
              frame 8 {
              }
              frame 9 {
              }
              frame 10 {
              }
              frame 11 {
              }
              frame 12 {
              }
              frame 13 {
              }
              frame 14 {
              }
              frame 15 {
              }
              frame 16 {
              }
              frame 17 {
              }
              frame 18 {
              }
              frame 19 {
              }
              frame 20 {
              }
              frame 21 {
              }
              frame 22 {
              }
              frame 23 {
              }
              frame 24 {
              }
              frame 25 {
              }
              frame 26 {
              }
              frame 27 {
              }
              frame 28 {
              }
              frame 29 {
              }
              frame 30 {
              }
              frame 31 {
              }
              frame 32 {
              }
              frame 33 {
              }
              frame 34 {
              }
              frame 35 {
              }
              frame 36 {
              }
            }
            n226 = case shown="3, 92" w387 {
              tunnel: ["总磷" ("table输入") "氨氮" ("table输入") "总氮" ("table输入")] -> w383
              frame 1, 131 {
              }
              frame 3, 92 {
              }
              frame 2, 76, Default {
              }
            }
            n227 = Get Date/Time In Seconds() -> (seconds since 1Jan1904=w384:timestamp)
            n228 = Bundle By Name(cluster=T17 {"时间标识"=timestamp(0 s since 1904-01-01), "设备"="", "日志信息"=""} ("data in"), "时间标识"=w384, "设备"=w383, "日志信息"=w382) -> (w385:T17)
            n229 = call "总氮报警信息.vi"("data in"=w385) -> ()  [unwired: 10 in, 1 out]
          }
        }
      }
    }
  }
  n230 = Bundle("参数下拉列表"=w5, "测量模式下拉列表"=w4, "量程下拉列表"=w3) -> (w2:T19)  [unwired: 1 in]
  n231 = property on="曲线模型" class="曲线模型 (严格)"("属性"=w2) -> (error out=w10:errorcluster)  [unwired: 2 in, 1 out]
  n232 = control-ref of="测量模式下拉列表"() -> (w16:refnum<vi>)
  n233 = control-ref of="量程参数读取"() -> (w6:refnum<vi>)
  n234 = control-ref of="参数下拉列表"() -> (w17:refnum<vi>)
  n235 = control-ref of="量程下拉列表"() -> (w18:refnum<vi>)
  n236 = Obtain Queue(name (unnamed)="TN" ("名称（未命名）"), element data type=cluster{"命令":string, "data":variant} {"命令"="", "data"=variant}) -> (queue out=w19:refnum<queue>, error out=w20:errorcluster)  [unwired: 3 in, 1 out]
  n237 = control-ref of="公式"() -> (w15:refnum<vi>)
  n238 = Obtain Notifier(name (unnamed)="TN" ("名称（未命名）"), notification data type=FALSE) -> (notifier out=w7:refnum<notifier>)  [unwired: 2 in, 2 out]
  n239 = while {
    tunnel: w19 -> [w466]
    tunnel: w20 -> [_]
    stop <- FALSE stop-if-true
    n240 = Get Queue Status(queue=w466) -> (queue out=w462:refnum<queue>, # elements in queue=w461:i32)  [unwired: 2 in, 6 out]
    n241 = Wait (ms)(milliseconds to wait=u32 1000 ("等待时间（毫秒）")) -> ()  [unwired: 1 out]
    n242 = case shown="0" w461 {
      tunnel: w462 -> [_ w469]
      frame Default {
      }
      frame 0 {
        w478 = u16 2 items=["总磷"=1, "总氮"=2, "氨氮"=3] ("站号")
        # "试剂填充 172 \n管路清洗108\n氨氮92\n总磷131\n总磷海水147\n总氮76\n总氮海水92"
        n243 = Bundle By Name(cluster=cluster{"命令":string, "data":variant} {"命令"="", "data"=variant} ("元素"), "命令"="读状态告警区", "data"=w478) -> (w484:cluster{"命令":string, "data":variant})
        n244 = Bundle By Name(cluster=cluster{"命令":string, "data":variant} {"命令"="", "data"=variant} ("元素"), "命令"="读测量数据区", "data"=w478) -> (w481:cluster{"命令":string, "data":variant})
        n245 = global read "VAR总氮全局变量.vi" "状态告警区"() -> (w470:T4)
        n246 = Unbundle By Name(w470) -> ("系统时间"=w477:timestamp)
        n247 = Enqueue Element(queue=w469, element=w484) -> (queue out=w479:refnum<queue>)  [unwired: 2 in, 2 out]
        n248 = Get Date/Time In Seconds() -> (seconds since 1Jan1904=w476:timestamp)
        n249 = Subtract(x=w476, y=w477) -> (x-y=w475:dbl)
        n250 = Absolute Value(x=w475) -> (abs(x)=w474:dbl)
        n251 = Enqueue Element(queue=w479, element=w481) -> (queue out=w471:refnum<queue>)  [unwired: 2 in, 2 out]
        n252 = Greater Or Equal?(x=w474, y=120.0) -> (x >= y?=w472:bool)
        n253 = case shown="真" w472 {
          tunnel: w471 -> [_ w487]
          frame False {
          }
          frame True {
            n254 = call "总氮启动命令.vi"("参数"=T20 {"站号"=3, "量程切换"=enum."AUTO", "控制命令"=enum."校时", "模式设置"=enum."待机", "测量间隔"=0}) -> ("启动命令"=w486:cluster{"命令":string, "data":variant})  [unwired: 10 in]
            n255 = Enqueue Element(queue=w487, element=w486) -> ()  [unwired: 2 in, 3 out]
          }
        }
      }
    }
    n256 = global read "总氮断电保存全局变量.vi" "流程路径"() -> (w465:path)
    n257 = global read "总氮断电保存全局变量.vi" "MB通信方式选择"() -> (w463:enum16{"串口", "TCP"})
    n258 = local write "流程路径"(w465) -> ()
    n259 = case shown="\"TCP\"" w463 {
      tunnel: [w489 w490] -> w464
      frame "串口", Default {
        n260 = global read "总氮断电保存全局变量.vi" "VISA Resource"() -> (w489:refnum<visa-resource-name>)
      }
      frame "TCP" {
        n261 = global read "总氮断电保存全局变量.vi" "IP"() -> (w490:string)
      }
    }
    "字符串" <- w464
  }
  n262 = while {
    tunnel: w19 -> [w497]
    tunnel: w18 -> [w496]
    tunnel: w17 -> [w495]
    tunnel: w16 -> [w494]
    tunnel: w15 -> [w493]
    tunnel: w6 -> [w492]
    tunnel: w10 -> [_]
    tunnel: w7 -> [w491]
    stop <- FALSE stop-if-true
    n263 = event shown="[2] \"布尔\": 鼠标按下" {
      selector: _ -> [_ _ _ _ _ _ _ _ _ _ _ _ _ _ _ _ _ _ _ _ _ _ _]
      dyn-events: _ -> [_ _ _ _ _ _ _ _ _ _ _ _ _ _ _ _ _ _ _ _ _ _ _]
      timeout: _ -> [_ _ _ _ _ _ _ _ _ _ _ _ _ _ _ _ _ _ _ _ _ _ _]
      tunnel: w497 -> [_ _ _ _ w517 w545 _ _ _ _ _ _ w647 _ w672 w679 _ _ _ _ _ _ _]
      tunnel: w496 -> [_ _ _ _ _ _ _ _ _ _ _ _ _ _ _ _ _ _ _ w695 _ _ _]
      tunnel: w495 -> [_ _ _ _ _ _ _ _ _ _ _ _ _ _ _ _ _ _ _ w693 _ w711 w718]
      tunnel: w494 -> [_ _ _ _ _ _ _ _ _ _ _ _ _ _ _ _ _ _ _ w694 _ _ _]
      tunnel: w493 -> [_ _ _ _ _ _ _ _ _ _ _ _ _ _ _ _ _ _ _ w689 _ _ _]
      tunnel: w492 -> [_ _ _ _ _ _ _ _ _ _ _ _ _ _ _ _ _ _ _ _ _ w709 _]
      tunnel: w491 -> [_ _ _ _ _ _ _ _ _ _ _ _ _ _ _ w675 _ _ _ _ _ _ _]
      tunnel: [_ _ _ w503 _ _ _ _ _ _ _ _ _ _ _ _ _ _ _ _ _ _ _] -> _
      event Timeout {
        n264 = event-data() -> ()  [unwired: 1 in, 3 out]
      }
      event "流程固件": Value Change {
        n265 = event-data() -> ()  [unwired: 1 in, 6 out]
        n266 = call "流程固件设置对话框.vi"() -> ()  [unwired: 12 in]
      }
      event "布尔": Mouse Down {
        n267 = event-data() -> ("CtlRef"=w500:refnum<vi>)  [unwired: 1 in, 5 out]
        n268 = property class="Bool (严格)"(reference=w500) -> ("Value"=w499:bool)  [unwired: 1 in, 2 out]
        n269 = case shown="假" w499 {
          frame False {
            n270 = call "密码键盘.vi"() -> ("NewNumber"=→"输入密码":dbl)  [unwired: 1 in]
          }
          frame True {
            n271 = local write "输入密码"(u32 0 ("输入密码")) -> ()
          }
        }
      }
      event "测量模式下拉列表", "量程下拉列表", "参数下拉列表": Value Change {
        n272 = event-data() -> ()  [unwired: 1 in, 6 out]
        n273 = local read "测量模式下拉列表"() -> (w505:enum16{"水样测量", "零点核查", "跨度核查", "标样核查", "加标回收"})
        n274 = local read "参数下拉列表"() -> (w504:enum16{"总磷", "总氮"})
        n275 = local read "量程下拉列表"() -> (w506:enum16{"低量程", "高量程"})
        n276 = Bundle("参数下拉列表"=w504, "测量模式下拉列表"=w505, "量程下拉列表"=w506) -> (w507:T19)  [unwired: 1 in]
        n277 = property on="曲线模型" class="曲线模型 (严格)"("属性"=w507) -> (error out=w503:errorcluster)  [unwired: 2 in, 1 out]
      }
      event "串口设置": Value Change {
        n278 = event-data() -> ()  [unwired: 1 in, 6 out]
        n279 = global read "总氮断电保存全局变量.vi" "MB通信方式选择"() -> (w508:enum16{"串口", "TCP"})
        n280 = global read "总氮断电保存全局变量.vi" "VISA Resource"() -> (w514:refnum<visa-resource-name>)
        n281 = global read "总氮断电保存全局变量.vi" "PORT"() -> (w513:string)
        n282 = global read "总氮断电保存全局变量.vi" "IP"() -> (w509:string)
        n283 = call "串口配置.vi"("PORT"=w513, "IP"=w509, "MB通信方式选择"=w508, "请选择串口:"=w514) -> ("PORT 2"=w511:string, "IP 2"=w512:string, "确认 2"=w515:bool, "VISA资源名称 2"=w516:refnum<visa-resource-name>, "MB通信方式选择 2"=w510:enum16{"串口", "TCP"})  [unwired: 3 in]
        n284 = case shown="真" w515 {
          tunnel: w516 -> [_ w522]
          tunnel: w517 -> [_ w521]
          tunnel: w512 -> [_ w520]
          tunnel: w511 -> [_ w519]
          tunnel: w510 -> [_ w518]
          frame False {
          }
          frame True {
            n285 = flat-sequence {
              tunnel: w522 -> [w527]
              tunnel: w521 -> [w528]
              tunnel: w520 -> [w526]
              tunnel: w519 -> [w525]
              tunnel: w518 -> [w524]
              frame #0 {
                n286 = global write "总氮断电保存全局变量.vi" "IP"(w526) -> ()
                n287 = global write "总氮断电保存全局变量.vi" "PORT"(w525) -> ()
                n288 = global write "总氮断电保存全局变量.vi" "VISA Resource"(w527) -> ()
                n289 = global write "总氮断电保存全局变量.vi" "MB通信方式选择"(w524) -> ()
                n290 = Flush Queue(queue=w528) -> (queue out=w523:refnum<queue>)  [unwired: 1 in, 2 out]
                n291 = Enqueue Element(queue=w523, element=cluster{"命令":string, "data":variant} {"命令"="启用模块", "data"=variant} ("元素")) -> ()  [unwired: 2 in, 3 out]
              }
              frame #1 {
                n292 = call <vilib>:"Application Directory.vi"() -> ("Application Directory"=w543:path)
                n293 = Build Path(base path=w543, name or relative path="data\\sys.ini" ("名称或相对路径")) -> (appended path=w541:path)
                n294 = call <vilib>:"Open Config Data.vi"("configuration file path"=w541) -> ("error out"=w537:errorcluster, "refnum"=w540:T13)  [unwired: 8 in, 1 out]
                n295 = vi-ref "总氮断电保存全局变量.vi"() -> (w539:refnum<vi>)
                n296 = call <userlib>:"Write Panel to INI__ogtk.vi"("error in (no error)"=w537, "VI ref"=w539, "refnum"=w540) -> ("error out"=w536:errorcluster, "refnum out"=w538:T13)  [unwired: 7 in]
                n297 = call <vilib>:"Close Config Data.vi"("error in (no error)"=w536, "refnum"=w538) -> ("error out"=w531:errorcluster, "file path"=w530:path)  [unwired: 8 in]
                n298 = Open/Create/Replace File(file path (use dialog)=w530, error in=w531) -> (refnum out=w534:refnum<file>, error out=w535:errorcluster)  [unwired: 4 in, 1 out]
                n299 = Flush File(refnum=w534, error in=w535) -> (refnum out=w533:refnum<file>, error out=w532:errorcluster)
                n300 = Close File(refnum=w533, error in=w532) -> ()  [unwired: 2 out]
              }
            }
          }
        }
      }
      event "模块启用": Value Change {
        n301 = event-data() -> ("OldVal"=w546:bool)  [unwired: 1 in, 5 out]
        n302 = Flush Queue(queue=w545) -> (queue out=w544:refnum<queue>)  [unwired: 1 in, 2 out]
        n303 = case shown="假" w546 {
          tunnel: w544 -> [w547 w549]
          frame False {
            n304 = Enqueue Element(queue=w547, element=cluster{"命令":string, "data":variant} {"命令"="停用模块", "data"=variant} ("元素")) -> ()  [unwired: 2 in, 3 out]
          }
          frame True {
            n305 = Enqueue Element(queue=w549, element=cluster{"命令":string, "data":variant} {"命令"="启用模块", "data"=variant} ("元素")) -> ()  [unwired: 2 in, 3 out]
          }
        }
      }
      event "流程路径": Value Change {
        n306 = event-data() -> ()  [unwired: 1 in, 6 out]
        n307 = flat-sequence {
          frame #0 {
            n308 = local read "流程路径"() -> (w551:path)
            n309 = global write "总氮断电保存全局变量.vi" "流程路径"(w551) -> ()
          }
          frame #1 {
            n310 = call <vilib>:"Application Directory.vi"() -> ("Application Directory"=w565:path)
            n311 = Build Path(base path=w565, name or relative path="data\\sys.ini" ("名称或相对路径")) -> (appended path=w563:path)
            n312 = call <vilib>:"Open Config Data.vi"("configuration file path"=w563) -> ("error out"=w559:errorcluster, "refnum"=w562:T13)  [unwired: 8 in, 1 out]
            n313 = vi-ref "总氮断电保存全局变量.vi"() -> (w561:refnum<vi>)
            n314 = call <userlib>:"Write Panel to INI__ogtk.vi"("error in (no error)"=w559, "VI ref"=w561, "refnum"=w562) -> ("error out"=w558:errorcluster, "refnum out"=w560:T13)  [unwired: 7 in]
            n315 = call <vilib>:"Close Config Data.vi"("error in (no error)"=w558, "refnum"=w560) -> ("error out"=w553:errorcluster, "file path"=w552:path)  [unwired: 8 in]
            n316 = Open/Create/Replace File(file path (use dialog)=w552, error in=w553) -> (refnum out=w556:refnum<file>, error out=w557:errorcluster)  [unwired: 4 in, 1 out]
            n317 = Flush File(refnum=w556, error in=w557) -> (refnum out=w555:refnum<file>, error out=w554:errorcluster)
            n318 = Close File(refnum=w555, error in=w554) -> ()  [unwired: 2 out]
          }
        }
      }
      event "公式一键写入": Value Change {
        n319 = event-data() -> ()  [unwired: 1 in, 6 out]
        n320 = local read "公式"() -> (w566:cluster{"X^2":dbl, "X":dbl, "b":dbl})
        n321 = call "公式复合写入.vi"("公式"=w566) -> ()  [unwired: 11 in]
      }
      event "曲线模型": Value Change {
        n322 = event-data() -> ()  [unwired: 1 in, 6 out]
        n323 = local write "公式"("曲线模型") -> ()
      }
      event "质控参数设置": Value Change {
        n324 = event-data() -> ()  [unwired: 1 in, 6 out]
        n325 = global read "总氮断电保存全局变量.vi" "质控参数设置"() -> (w568:T21)
        n326 = call "总氮质控参数设置.vi"("质控参数设置"=w568) -> ("输出簇"=w569:T22)  [unwired: 10 in]
        n327 = Unbundle By Name(w569) -> ("确定"=w570:bool)
        n328 = case shown="真" w570 {
          tunnel: w569 -> [_ w572]
          tunnel: w568 -> [_ w571]
          frame False {
          }
          frame True {
            n329 = flat-sequence {
              tunnel: w572 -> [w579]
              tunnel: w571 -> [w578]
              frame #0 {
                n330 = Unbundle By Name(w579) -> ("跨度值"=w577:dbl, "零点标准液浓度"=w576:dbl, "跨度标准液浓度"=w575:dbl, "标准液标准浓度"=w574:dbl)
                n331 = Bundle By Name(cluster=w578, "跨度值"=w577, "零点标准液浓度"=w576, "跨度标准液浓度"=w575, "标准液标准浓度"=w574) -> (w573:T21)
                n332 = global write "总氮断电保存全局变量.vi" "质控参数设置"(w573) -> ()
              }
              frame #1 {
                n333 = call <vilib>:"Application Directory.vi"() -> ("Application Directory"=w593:path)
                n334 = Build Path(base path=w593, name or relative path="data\\sys.ini" ("名称或相对路径")) -> (appended path=w591:path)
                n335 = call <vilib>:"Open Config Data.vi"("configuration file path"=w591) -> ("error out"=w587:errorcluster, "refnum"=w590:T13)  [unwired: 8 in, 1 out]
                n336 = vi-ref "总氮断电保存全局变量.vi"() -> (w589:refnum<vi>)
                n337 = call <userlib>:"Write Panel to INI__ogtk.vi"("error in (no error)"=w587, "VI ref"=w589, "refnum"=w590) -> ("error out"=w586:errorcluster, "refnum out"=w588:T13)  [unwired: 7 in]
                n338 = call <vilib>:"Close Config Data.vi"("error in (no error)"=w586, "refnum"=w588) -> ("error out"=w581:errorcluster, "file path"=w580:path)  [unwired: 8 in]
                n339 = Open/Create/Replace File(file path (use dialog)=w580, error in=w581) -> (refnum out=w584:refnum<file>, error out=w585:errorcluster)  [unwired: 4 in, 1 out]
                n340 = Flush File(refnum=w584, error in=w585) -> (refnum out=w583:refnum<file>, error out=w582:errorcluster)
                n341 = Close File(refnum=w583, error in=w582) -> ()  [unwired: 2 out]
              }
            }
          }
        }
      }
      event "仪器参数设置": Value Change {
        n342 = event-data() -> ()  [unwired: 1 in, 6 out]
        n343 = global read "总氮断电保存全局变量.vi" "总氮仪器参数"() -> (w594:T23)
        n344 = call "仪器参数设置.vi"("仪器参数设置"=w594) -> ("仪器参数设置输出"=w595:T24)  [unwired: 10 in]
        n345 = Unbundle By Name(w595) -> ("确定"=w596:bool)
        n346 = case shown="真" w596 {
          tunnel: w595 -> [_ w598]
          tunnel: w594 -> [_ w597]
          frame False {
          }
          frame True {
            n347 = flat-sequence {
              tunnel: w598 -> [w615]
              tunnel: w597 -> [w614]
              frame #0 {
                n348 = Unbundle By Name(w615) -> ("测量量程"=w613:dbl, "测量精度"=w612:dbl, "测量间隔"=w611:dbl, "消解温度"=w610:dbl, "消解时长"=w608:dbl, "空白校准时间"=w607:timestamp, "曲线截距"=w606:dbl, "曲线斜率"=w605:dbl, "测量检出限"=w604:dbl, "测量信号值"=w603:dbl, "线性相关系数"=w602:dbl, "二次多项式系数"=w601:dbl, "标样校准时间"=w600:timestamp, "单位"=w599:u16)
                n349 = Bundle By Name(cluster=w614, "测量量程"=w613, "测量精度"=w612, "测量间隔"=w611, "消解温度"=w610, "消解时长"=w608, "空白校准时间"=w607, "曲线截距"=w606, "曲线斜率"=w605, "测量检出限"=w604, "测量信号值"=w603, "线性相关系数"=w602, "二次多项式系数"=w601, "标样校准时间"=w600, "单位"=w599) -> (w609:T23)
                n350 = global write "总氮断电保存全局变量.vi" "总氮仪器参数"(w609) -> ()
              }
              frame #1 {
                n351 = call <vilib>:"Application Directory.vi"() -> ("Application Directory"=w629:path)
                n352 = Build Path(base path=w629, name or relative path="data\\sys.ini" ("名称或相对路径")) -> (appended path=w627:path)
                n353 = call <vilib>:"Open Config Data.vi"("configuration file path"=w627) -> ("error out"=w623:errorcluster, "refnum"=w626:T13)  [unwired: 8 in, 1 out]
                n354 = vi-ref "总氮断电保存全局变量.vi"() -> (w625:refnum<vi>)
                n355 = call <userlib>:"Write Panel to INI__ogtk.vi"("error in (no error)"=w623, "VI ref"=w625, "refnum"=w626) -> ("error out"=w622:errorcluster, "refnum out"=w624:T13)  [unwired: 7 in]
                n356 = call <vilib>:"Close Config Data.vi"("error in (no error)"=w622, "refnum"=w624) -> ("error out"=w617:errorcluster, "file path"=w616:path)  [unwired: 8 in]
                n357 = Open/Create/Replace File(file path (use dialog)=w616, error in=w617) -> (refnum out=w620:refnum<file>, error out=w621:errorcluster)  [unwired: 4 in, 1 out]
                n358 = Flush File(refnum=w620, error in=w621) -> (refnum out=w619:refnum<file>, error out=w618:errorcluster)
                n359 = Close File(refnum=w619, error in=w618) -> ()  [unwired: 2 out]
              }
            }
          }
        }
      }
      event "自动测试量程配置": Value Change {
        n360 = event-data() -> ()  [unwired: 1 in, 6 out]
        n361 = flat-sequence {
          frame #0 {
            n362 = global write "总氮断电保存全局变量.vi" "总氮自动测试量程配置"("自动测试量程配置") -> ()
          }
          frame #1 {
            n363 = call <vilib>:"Application Directory.vi"() -> ("Application Directory"=w644:path)
            n364 = Build Path(base path=w644, name or relative path="data\\sys.ini" ("名称或相对路径")) -> (appended path=w642:path)
            n365 = call <vilib>:"Open Config Data.vi"("configuration file path"=w642) -> ("error out"=w638:errorcluster, "refnum"=w641:T13)  [unwired: 8 in, 1 out]
            n366 = vi-ref "总氮断电保存全局变量.vi"() -> (w640:refnum<vi>)
            n367 = call <userlib>:"Write Panel to INI__ogtk.vi"("error in (no error)"=w638, "VI ref"=w640, "refnum"=w641) -> ("error out"=w637:errorcluster, "refnum out"=w639:T13)  [unwired: 7 in]
            n368 = call <vilib>:"Close Config Data.vi"("error in (no error)"=w637, "refnum"=w639) -> ("error out"=w632:errorcluster, "file path"=w631:path)  [unwired: 8 in]
            n369 = Open/Create/Replace File(file path (use dialog)=w631, error in=w632) -> (refnum out=w635:refnum<file>, error out=w636:errorcluster)  [unwired: 4 in, 1 out]
            n370 = Flush File(refnum=w635, error in=w636) -> (refnum out=w634:refnum<file>, error out=w633:errorcluster)
            n371 = Close File(refnum=w634, error in=w633) -> ()  [unwired: 2 out]
          }
        }
      }
      event "手动启动": Value Change {
        n372 = event-data() -> ()  [unwired: 1 in, 6 out]
        n373 = call "总氮启动参数对话框.vi"() -> ("确认"=w645:bool, "元素"=w646:cluster{"命令":string, "data":variant})  [unwired: 10 in]
        n374 = case shown="真" w645 {
          tunnel: w647 -> [_ w649]
          tunnel: w646 -> [_ w648]
          frame False {
          }
          frame True {
            n375 = Enqueue Element(queue=w649, element=w648) -> ()  [unwired: 2 in, 3 out]
          }
        }
      }
      event "定时启动": Mouse Down {
        n376 = event-data() -> ()  [unwired: 1 in, 6 out]
        n377 = flat-sequence {
          frame #0 {
            n378 = global read "总氮断电保存全局变量.vi" "定时控制"() -> (w651:T6)
            n379 = call "总氮周期设置.vi"("定时控制输入"=w651) -> ("定时控制输出"=w650:T25)  [unwired: 10 in]
            n380 = global write "总氮断电保存全局变量.vi" "定时控制"(w650) -> ()
          }
          frame #1 {
            n381 = call <vilib>:"Application Directory.vi"() -> ("Application Directory"=w665:path)
            n382 = Build Path(base path=w665, name or relative path="data\\sys.ini" ("名称或相对路径")) -> (appended path=w663:path)
            n383 = call <vilib>:"Open Config Data.vi"("configuration file path"=w663) -> ("error out"=w659:errorcluster, "refnum"=w662:T13)  [unwired: 8 in, 1 out]
            n384 = vi-ref "总氮断电保存全局变量.vi"() -> (w661:refnum<vi>)
            n385 = call <userlib>:"Write Panel to INI__ogtk.vi"("error in (no error)"=w659, "VI ref"=w661, "refnum"=w662) -> ("error out"=w658:errorcluster, "refnum out"=w660:T13)  [unwired: 7 in]
            n386 = call <vilib>:"Close Config Data.vi"("error in (no error)"=w658, "refnum"=w660) -> ("error out"=w653:errorcluster, "file path"=w652:path)  [unwired: 8 in]
            n387 = Open/Create/Replace File(file path (use dialog)=w652, error in=w653) -> (refnum out=w656:refnum<file>, error out=w657:errorcluster)  [unwired: 4 in, 1 out]
            n388 = Flush File(refnum=w656, error in=w657) -> (refnum out=w655:refnum<file>, error out=w654:errorcluster)
            n389 = Close File(refnum=w655, error in=w654) -> ()  [unwired: 2 out]
          }
        }
      }
      event "单步测试": Value Change {
        w667 = u16 1 items=["总磷"=1, "氨氮"=3] ("站号")
        n390 = event-data() -> ()  [unwired: 1 in, 6 out]
        n391 = Bundle("站号"=w667, "总磷氨氮调试"="总磷氨氮调试") -> (w666:cluster{"站号":u16, "总磷氨氮调试":u16[]})  [unwired: 1 in]
        n392 = Bundle By Name(cluster=cluster{"命令":string, "data":variant} {"命令"="", "data"=variant} ("元素"), "命令"="debug", "data"=w666) -> (w669:cluster{"命令":string, "data":variant})
        n393 = Enqueue Element(queue=w672, element=w669) -> ()  [unwired: 2 in, 3 out]
      }
      event "停止": Value Change {
        n394 = event-data() -> ()  [unwired: 1 in, 6 out]
        n395 = Enqueue Element(queue=w679, element=cluster{"命令":string, "data":variant} {"命令"="启动", "data"=variant(cluster{"站号":u16, "控制命令输出":u16[]} {"站号"=1, "控制命令输出"=[2816]})} ("元素")) -> (queue out=w676:refnum<queue>)  [unwired: 2 in, 2 out]
        n396 = Cancel Notification(0:w675) -> (8:w674:refnum<notifier>)  [unwired: 1 in, 2 out]
        n397 = Send Notification(notification=TRUE ("通知"), notifier=w674) -> ()  [unwired: 1 in, 2 out]
        n398 = Enqueue Element(queue=w676, element=cluster{"命令":string, "data":variant} {"命令"="启动", "data"=variant(cluster{"站号":u16, "控制命令输出":u16[]} {"站号"=2, "控制命令输出"=[2816]})} ("元素")) -> ()  [unwired: 2 in, 3 out]
      }
      event "设置": Value Change {
        n399 = event-data() -> ()  [unwired: 1 in, 6 out]
        n400 = property on="窗格" class="Pane"("Origin"=T11 {"Horizontal"=0, "Vertical"=628} ("原点")) -> ()  [unwired: 2 in, 2 out]
      }
      event "返回": Value Change {
        n401 = event-data() -> ()  [unwired: 1 in, 6 out]
        n402 = property on="窗格" class="Pane"("Origin"=T11 {"Horizontal"=0, "Vertical"=0} ("原点")) -> ()  [unwired: 2 in, 2 out]
      }
      event "公式.X^2", "公式.X", "公式.b": Mouse Down {
        n403 = event-data() -> ("CtlRef"=w685:refnum<vi>)  [unwired: 1 in, 5 out]
        n404 = property class="DigNum (严格)"(reference=w685) -> (reference out=w683:refnum<vi>, "Value"=w684:dbl)  [unwired: 1 in, 1 out]
        n405 = call "数字键盘.vi"("OldNumber"=w684) -> ("NewNumber"=w682:dbl)
        n406 = property class="DigNum (严格)"(reference=w683, "Val(Sgnl)"=w682) -> ()  [unwired: 1 in, 2 out]
      }
      event "读公式": Value Change {
        n407 = event-data() -> ()  [unwired: 1 in, 6 out]
        n408 = property class="Enum (严格)"(reference=w693) -> ("Value"=w692:enum16{"总磷", "总氮"})  [unwired: 1 in, 2 out]
        n409 = property class="Enum (严格)"(reference=w694) -> ("Value"=w691:enum16{"水样测量", "零点核查", "跨度核查", "标样核查", "加标回收"})  [unwired: 1 in, 2 out]
        n410 = property class="Enum (严格)"(reference=w695) -> ("Value"=w690:enum16{"低量程", "高量程"})  [unwired: 1 in, 2 out]
        n411 = call "总磷总氮公式读取.vi"("量程"=w690, "测量模式"=w691, "测量参数"=w692) -> ("error out"=w687:errorcluster, "公式"=w688:cluster{"X^2":dbl, "X":dbl, "b":dbl})  [unwired: 7 in]
        n412 = property class="Clust (严格)"(reference=w689, "Value"=w688) -> ()  [unwired: 1 in, 2 out]
        n413 = case shown="错误" w687 {
          tunnel: ["读取成功" ("消息") "读取失败" ("消息")] -> w686
          frame No Error {
          }
          frame Error {
          }
        }
        n414 = One Button Dialog(message=w686) -> ()  [unwired: 1 in, 1 out]
      }
      event "写公式": Value Change {
        n415 = event-data() -> ()  [unwired: 1 in, 6 out]
        n416 = call "总磷总氮公式写入.vi"("公式"="公式", "量程"="量程下拉列表", "测量模式"="测量模式下拉列表", "测量参数"="参数下拉列表") -> ("error out"=w700:errorcluster)  [unwired: 7 in]
        n417 = case shown="无错误" w700 {
          tunnel: ["写入成功" ("消息") "写入失败" ("消息")] -> w701
          frame No Error {
          }
          frame Error {
          }
        }
        n418 = One Button Dialog(message=w701) -> ()  [unwired: 1 in, 1 out]
      }
      event "量程切换阈值读取": Value Change {
        n419 = event-data() -> ()  [unwired: 1 in, 6 out]
        n420 = property class="Enum (严格)"(reference=w711) -> ("Value"=w710:enum16{"总磷", "总氮"})  [unwired: 1 in, 2 out]
        n421 = call "总磷总氮量程读取.vi"("测量参数"=w710) -> ("error out"=w706:errorcluster, "量程参数读取"=w708:T26)  [unwired: 9 in]
        n422 = property class="Clust (严格)"(reference=w709, "Value"=w708) -> ()  [unwired: 1 in, 2 out]
        n423 = case shown="错误" w706 {
          tunnel: ["读取成功" ("消息") "读取失败" ("消息")] -> w707
          frame No Error {
          }
          frame Error {
          }
        }
        n424 = One Button Dialog(message=w707) -> ()  [unwired: 1 in, 1 out]
      }
      event "量程切换阈值写入": Value Change {
        n425 = event-data() -> ()  [unwired: 1 in, 6 out]
        n426 = property class="Enum (严格)"(reference=w718) -> ("Value"=w717:enum16{"总磷", "总氮"})  [unwired: 1 in, 2 out]
        n427 = call "总磷总氮量程写入.vi"("量程参数写入"="量程参数读取", "测量参数"=w717) -> ("error out"=w715:errorcluster)  [unwired: 8 in]
        n428 = case shown="无错误" w715 {
          tunnel: ["写入成功" ("消息") "写入失败" ("消息")] -> w716
          frame No Error {
          }
          frame Error {
          }
        }
        n429 = One Button Dialog(message=w716) -> ()  [unwired: 1 in, 1 out]
      }
    }
  }
